vi "Encoder.vi"(9 "B Channel":T1=enum."DIO 1", 11 "A Channel":T1) -> (1 "Distance":dbl, 3 "Rate":dbl)   [LabVIEW 2025]
uses:
  <vilib>/Rock Robotics/SystemInterfaces/DIO/FPGA_DIOChannel.ctl
  <vilib>/Rock Robotics/WPI/Counter/WPI_CounterDigitalInputToDigitalSource.vi
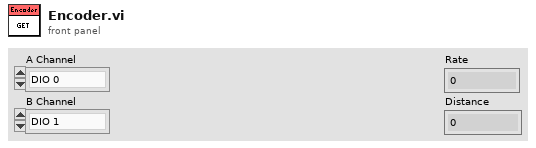
[diagram p1: front panel]
types:
  T1 = typedef "FPGA_DIOChannel.ctl" = enum8{"DIO 0", "DIO 1", "DIO 2", "DIO 3", "DIO 4", "DIO 5", "DIO 6", "DIO 7", "DIO 8", "DIO 9", "DIO MXP 0", "DIO MXP 1", "DIO MXP 2", "DIO MXP 3", "DIO MXP 4", "DIO MXP 5", "DIO MXP 6", "DIO MXP 7", "DIO MXP 8", "DIO MXP 9", "DIO MXP 10", "DIO MXP 11", "DIO MXP 12", "DIO MXP 13", "DIO MXP 14", "DIO MXP 15", "SPI Port CS1", "SPI Port CS2", "SPI Port CS3", "SPI Port MISO", "SPI Port MOSI", "Invalid"}
  T2 = typedef "WPI_EncoderDevRef.ctl" = cluster{"DevStatus":errorcluster, "EncoderIndex":T3, "CounterIndex":T4, "DistancePerCount":dbl, "Decoding Type":T5}
  T3 = typedef "FPGA_EncoderIdx.ctl" = enum8{"Enc 0", "Enc 1", "Enc 2", "Enc 3", "Enc 4", "Enc 5", "Enc 6", "Enc 7", "Invalid"}
  T4 = typedef "FPGA_CounterCtrSystemIndex.ctl" = enum8{"Ctr 0", "Ctr 1", "Ctr 2", "Ctr 3", "Ctr 4", "Ctr 5", "Ctr 6", "Ctr 7", "Invalid"}
  T5 = typedef "WPI_EncoderType.ctl" = enum16{"1x", "2x", "4x"}
  T6 = typedef "WPI_DigitalInputDevRef.ctl" = cluster{"DevStatus":errorcluster, "DIO Channel":T1}
  T7 = typedef "FPGA_CounterEncoderSourceConvertionLVSourceType.ctl" = cluster{"DevStatus":errorcluster, "AnalogTriggerMode?":bool, "DigitalMode":cluster{"DIO Channel":T8}, "AnalogTriggerMode":cluster{"AnalogTriggerIndex":T9, "OutputType":T10}}
  T8 = typedef "FPGA_DIODigitalSourceChannel.ctl" = enum8{"DIO 0", "DIO 1", "DIO 2", "DIO 3", "DIO 4", "DIO 5", "DIO 6", "DIO 7", "DIO 8", "DIO 9", "DIO MXP 0", "DIO MXP 1", "DIO MXP 2", "DIO MXP 3", "DIO MXP 4", "DIO MXP 5", "DIO MXP 6", "DIO MXP 7", "DIO MXP 8", "DIO MXP 9", "DIO MXP 10", "DIO MXP 11", "DIO MXP 12", "DIO MXP 13", "DIO MXP 14", "DIO MXP 15", "SPI Port CS1", "SPI Port CS2", "SPI Port CS3", "SPI Port MISO", "SPI Port MOSI", "Disabled"}
  T9 = typedef "FPGA_AnalogTriggerIndex.ctl" = enum8{"Trig 0", "Trig 1", "Trig 2", "Trig 3", "Trig 4", "Trig 5", "Trig 6", "Trig 7", "Invalid"}
  T10 = typedef "FPGA_AnalogTriggerOutType.ctl" = enum16{"InWindow", "TriggerState", "Rising", "Falling"}
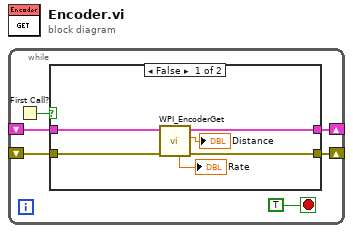
[diagram p0: block diagram]
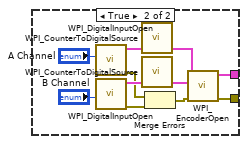
[diagram p2: hidden frame]
diagram:
  n1 = while {
    shift-right: [w4] -> _
    shift-left: _ -> [w1]
    shift-right: [w3] -> _
    shift-left: _ -> [w2]
    stop <- TRUE stop-if-true
    n2 = First Call?() -> (First Call?: T/F=w5:bool)
    n3 = case shown="False" w5 {
      tunnel: [w9 w14] -> w4
      tunnel: [w10 w13] -> w3
      tunnel: w2 -> [w12 _]
      tunnel: w1 -> [w11 _]
      frame False {
        n4 = call <vilib>:"WPI_EncoderGet.vi"("error in (no error)"=w11, "EncoderDevRef"=w12) -> ("error out"=w9:errorcluster, "Distance"=→"Distance":dbl, "EncoderDevRef"=w10:T2, "Rate"=→"Rate":dbl)  [unwired: 4 in, 2 out]
      }
      frame True {
        n5 = call <vilib>:"WPI_DigitalInputOpen.vi"("DIO Channel"="A Channel") -> ("error out"=w17:errorcluster, "DigitalInputDevRef"=w22:T6)  [unwired: 1 in, 8 out]
        n6 = call <vilib>:"WPI_DigitalInputOpen.vi"("DIO Channel"="B Channel") -> ("error out"=w16:errorcluster, "DigitalInputDevRef"=w21:T6)  [unwired: 1 in, 8 out]
        n7 = call-poly <vilib>:"WPI_CounterToDigitalSource.vi"("DigitalInputDevRef"=w22) -> ("Digital Source"=w23:T7)  [unwired: 6 out]
        n8 = call-poly <vilib>:"WPI_CounterToDigitalSource.vi"("DigitalInputDevRef"=w21) -> ("Digital Source"=w20:T7)  [unwired: 6 out]
        n9 = Merge Errors(w17, w16) -> (w15:errorcluster)
        n10 = call <vilib>:"WPI_EncoderOpen.vi"("error in (no error)"=w15, "BSource"=w20, "ASource"=w23) -> ("error out"=w14:errorcluster, "EncoderDevRef"=w13:T2)  [unwired: 5 in, 2 out]
      }
    }
  }
